vi "Write data.vi"(8 "error in (no error)":errorcluster, 10 "data":string, 11 "Object in":refnum<class "Object.lvclass">) -> (0 "error out":errorcluster, 3 "Object out":refnum<class "Object.lvclass">)   [LabVIEW 2015, in "NI_AWS_S3.lvlib" / "Object.lvclass"]
uses:
  Object.lvclass
  Object.lvclass/Object.ctl
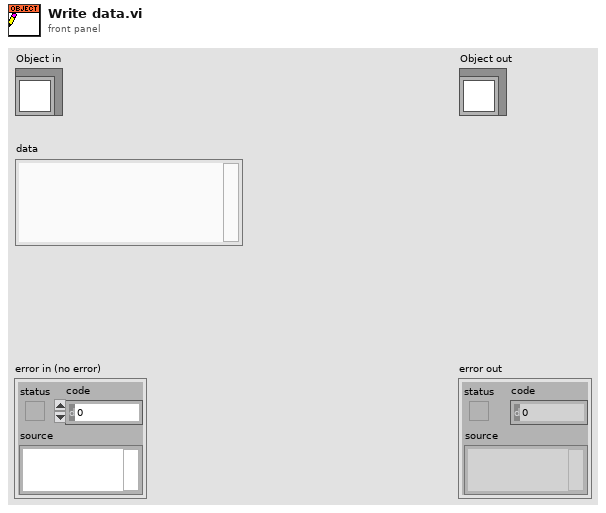
[diagram p1: front panel]
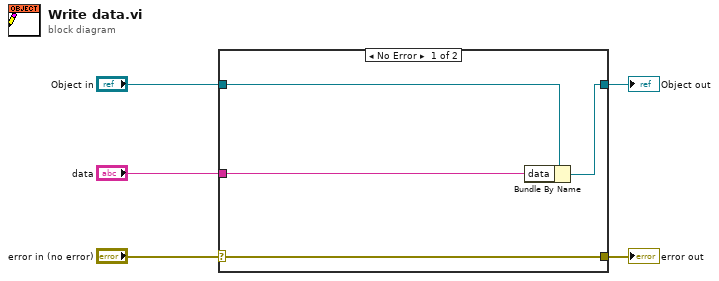
[diagram p0: block diagram]
diagram:
  n1 = case shown="No Error" "error in (no error)" {
    selector: "error in (no error)" -> [w9 w10]
    tunnel: [w9 w10] -> w4
    tunnel: [w7 w11] -> w2
    tunnel: "Object in" -> [w8 w11]
    tunnel: "data" -> [w6 _]
    frame No Error {
      n2 = Bundle By Name(cluster=w8, "data"=w6) -> (w7:refnum<class "Object.lvclass">)
    }
    frame Error {
    }
  }
  "error out" <- w4
  "Object out" <- w2
